vi "ArrayIntoString(SubVI).vi"(1 "Array":dbl[](array[numeric])) -> (0 "Result string":string)   [LabVIEW 2018]
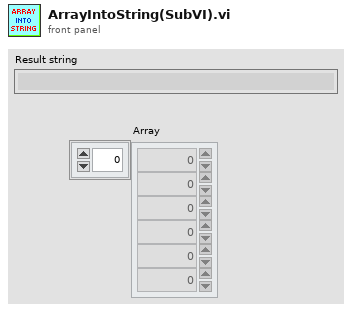
[diagram p1: front panel]
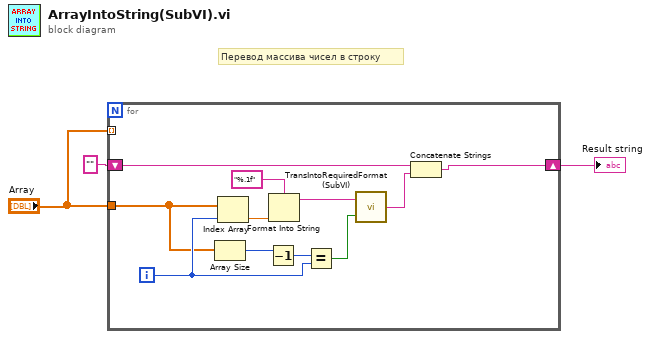
[diagram p0: block diagram]
diagram:
  # "Перевод массива чисел в строку"
  n1 = for {
    tunnel: "Array" -> [_] mode=indexing
    tunnel: "Array" -> [w4]
    shift-right: [w10] -> w3
    shift-left: "" -> [w13]
    i -> [w12]
    n2 = Array Size(array=w4) -> (size(s)=w9:i32)
    n3 = Index Array(array=w4, index=w12) -> (element=w14:dbl)
    n4 = Decrement(x=w9) -> (x-1=w8:i32)
    n5 = Format Into String(format string="%.1f", w14) -> (resulting string=w5:string)  [unwired: 2 in, 1 out]
    n6 = Equal?(x=w8, y=w12) -> (x = y?=w11:bool)
    n7 = call "TransIntoRequiredFormat(SubVI).vi"("Boolean"=w11, "String In"=w5) -> ("String Out"=w6:string)
    n8 = Concatenate Strings(w13, w6) -> (w10:string)
  }
  "Result string" <- w3
